vi "Test Lookup API.vi"() -> (0 "test result":errorcluster)   [LabVIEW 2014, in "LVCOOOP Tests.lvlib"]
uses:
  LVCOOOP Tests.lvlib
  Base Class A.lvclass
  Class B.lvclass
  Class C.lvclass
  LVCOOOP/Lookup API/Services/Lookup Service/Lookup Service.lvclass
panel:
  out "pass?":bool
  out "should be equal 2":bool
  out "should be equal 1":bool
  out "expect error 1446":errorcluster caption="expect error 1446 because attempt to add non-member child class"
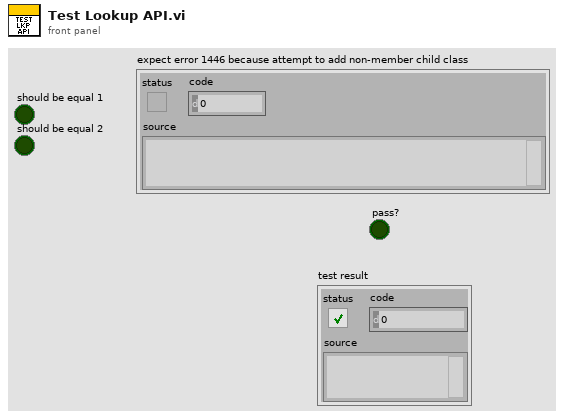
[diagram p1: front panel]
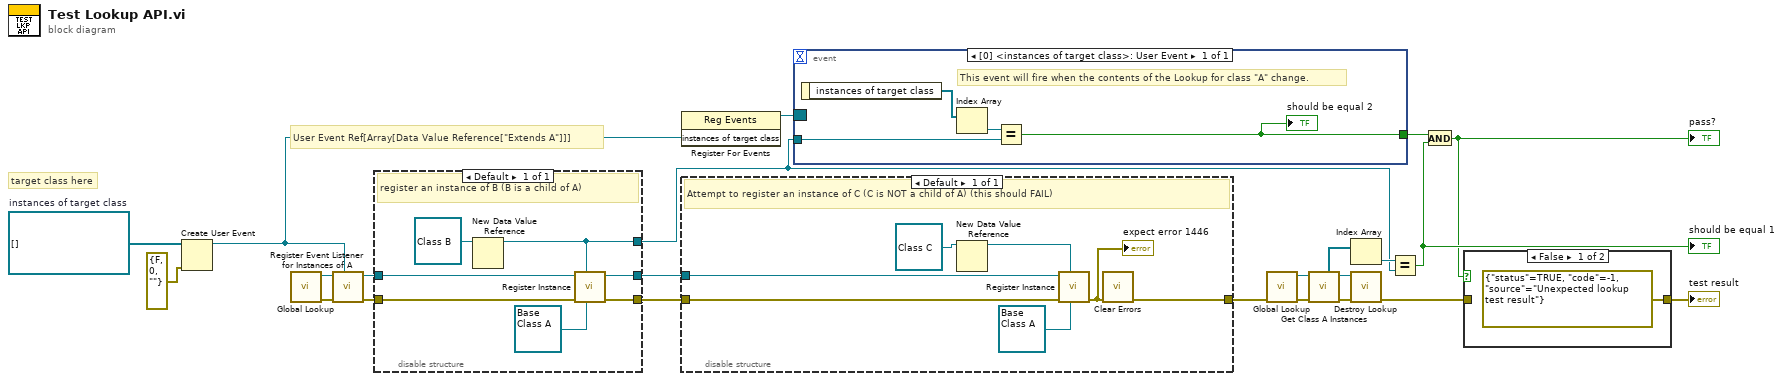
[diagram p0: block diagram]
diagram:
  w22 = refnum<data-value>[] []  # instances of target class
  # "User Event Ref[Array[Data Value Reference[\"Extends A\"]]]"
  # "target class here"
  n1 = Create User Event(user event datatype=w22, error in=errorcluster {"status"=FALSE, "code"=0, "source"=""} ("error in (no error)")) -> (user event=w7:refnum<user-event>)  [unwired: 1 out]
  n2 = call "Global Lookup.vi"() -> ("error out"=w4:errorcluster, "Global Lookup"=w5:refnum<data-value>)  [unwired: 10 in]
  n3 = call "Register Event Listener for Instances of A.vi"("class A instances event ref"=w7, "error in (no error)"=w4, "Lookup in"=w5) -> ("error out"=w9:errorcluster, "Lookup out"=w21:refnum<data-value>)  [unwired: 7 in]
  n4 = disable-structure shown="Default" {
    disable-tunnel: w21 -> [w29]
    disable-tunnel: [w28] -> w20
    disable-tunnel: [w24] -> w16
    disable-tunnel: w9 -> [w27]
    disable-tunnel: [w26] -> w8
    frame Enabled {
      # "register an instance of B (B is a child of A)"
      n5 = New Data Value Reference(data value=refnum<class "Class B.lvclass"> refnum ("LVCOOOP Tests.lvlib:Class B.lvclass")) -> (data value reference=w24:refnum<data-value>)  [unwired: 1 in, 1 out]
      n6 = call "Register Instance.vi"("Base Class (LabVIEW Object)"=refnum<class "Base Class A.lvclass"> refnum ("LVCOOOP Tests.lvlib:Base Class A.lvclass"), "Object Instance"=w24, "error in (no error)"=w27, "Lookup Service in"=w29) -> ("error out"=w26:errorcluster, "Lookup Service out"=w28:refnum<data-value>)  [unwired: 6 in]
    }
  }
  n7 = register-events(w7) -> (reference out=w23:refnum<event-registration>)  [unwired: 2 in, 1 out]
  n8 = disable-structure shown="Default" {
    disable-tunnel: w20 -> [w37]
    disable-tunnel: w8 -> [w35]
    disable-tunnel: [w31] -> w3
    frame Enabled {
      # "Attempt to register an instance of C (C is NOT a child of A) (this should FAIL)"
      n9 = New Data Value Reference(data value=refnum<class "Class C.lvclass"> refnum ("LVCOOOP Tests.lvlib:Class C.lvclass")) -> (data value reference=w33:refnum<data-value>)  [unwired: 1 in, 1 out]
      n10 = call "Register Instance.vi"("Base Class (LabVIEW Object)"=refnum<class "Base Class A.lvclass"> refnum ("LVCOOOP Tests.lvlib:Base Class A.lvclass"), "Object Instance"=w33, "error in (no error)"=w35, "Lookup Service in"=w37) -> ("error out"=w32:errorcluster)  [unwired: 6 in, 1 out]
      "expect error 1446" <- w32
      n11 = call <vilib>:"Clear Errors.vi"("error in (no error)"=w32) -> ("error out"=w31:errorcluster)  [unwired: 5 in, 1 out]
    }
  }
  n12 = event shown="[0] <instances of target class>: User Event" {
    selector: w23 -> [_]
    dyn-events: _ -> [_]
    timeout: _ -> [_]
    tunnel: w16 -> [w39]
    tunnel: [w38] -> w15
    event User Event {
      # "This event will fire when the contents of the Lookup for class \"A\" change."
      n13 = event-data() -> ("instances of target class"=w41:refnum<data-value>[])  [unwired: 1 in]
      n14 = Index Array(array=w41) -> (element=w40:refnum<data-value>)  [unwired: 1 in]
      n15 = Equal?(x=w40, y=w39) -> (x = y?=w38:bool)
      "should be equal 2" <- w38
    }
  }
  n16 = call "Global Lookup.vi"("error in (no error)"=w3) -> ("error out"=w2:errorcluster, "Global Lookup"=w1:refnum<data-value>)  [unwired: 9 in]
  n17 = call "Get Class A Instances.vi"("error in (no error)"=w2, "Lookup in"=w1) -> ("error out"=w17:errorcluster, "Lookup out"=w18:refnum<data-value>, "instances of A"=w6:refnum<data-value>[])  [unwired: 7 in]
  n18 = Index Array(array=w6) -> (element=w19:refnum<data-value>)  [unwired: 1 in]
  n19 = call "Destroy Lookup.vi"("error in (no error)"=w17, "Lookup Service in"=w18) -> ("error out"=w11:errorcluster)  [unwired: 9 in]
  n20 = Equal?(x=w19, y=w16) -> (x = y?=w14:bool)
  "should be equal 1" <- w14
  n21 = And(x=w15, y=w14) -> (x .and. y?=w13:bool)
  "pass?" <- w13
  n22 = case shown="False" w13 {
    tunnel: [errorcluster {"status"=TRUE, "code"=-1, "source"="Unexpected lookup test result"} ("test result") w43] -> w12
    tunnel: w11 -> [_ w43]
    frame False {
    }
    frame True {
    }
  }
  "test result" <- w12
